vi "Actor Core.vi"(8 "error in":errorcluster, 11 "Network Endpoint":refnum<class "Network Endpoint.lvclass">) -> (0 "error out":errorcluster, 3 "Actor out":refnum<class "Actor.lvclass">)   [LabVIEW 2020, in "Network Endpoint.lvlib" / "Network Endpoint.lvclass"]
doc: "Manages the reader network stream. Waits for a remote writer to connect. Once a connection is established, forwards received messages to its parent node."
uses:
  Network Endpoint.lvclass
  C:/Program Files (x86)/National Instruments/LabVIEW 2020/vi.lib/ActorFramework/Actor/Actor.lvclass
  <vilib>/ActorFramework/Actor/Actor.lvclass
  <vilib>/ActorFramework/Actor/Actor.lvclass/Actor.ctl
  <vilib>/ActorFramework/Message Enqueuer/Message Enqueuer.lvclass/Message Enqueuer.ctl
  Network Endpoint.lvclass/Network Endpoint.ctl
  <vilib>/ActorFramework/Report Error Msg/Report Error Msg.lvclass/Report Error Msg.ctl
  <vilib>/ActorFramework/Message Enqueuer/Init from Existing Queue.vi
  <vilib>/ActorFramework/Report Error Msg/Report Error Msg.lvclass
  C:/Program Files (x86)/National Instruments/LabVIEW 2020/vi.lib/ActorFramework/Message/Message.lvclass
  <vilib>/ActorFramework/Message Priority Queue/Priority Enqueue.vi
  Abstract Classes/Message Stream/Message Stream.lvclass
  <vilib>/ActorFramework/Message Enqueuer/Message Enqueuer.lvclass
  Abstract Classes/Message Flattener/Message Flattener.lvclass
  <resource>/AFDebug/AF Debug.lvlib
  <vilib>/ActorFramework/Message/Message.lvclass
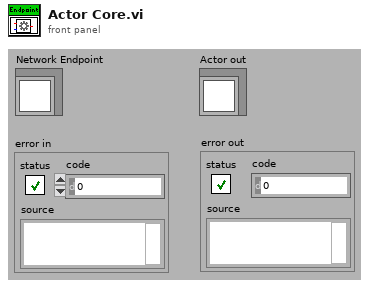
[diagram p1: front panel]
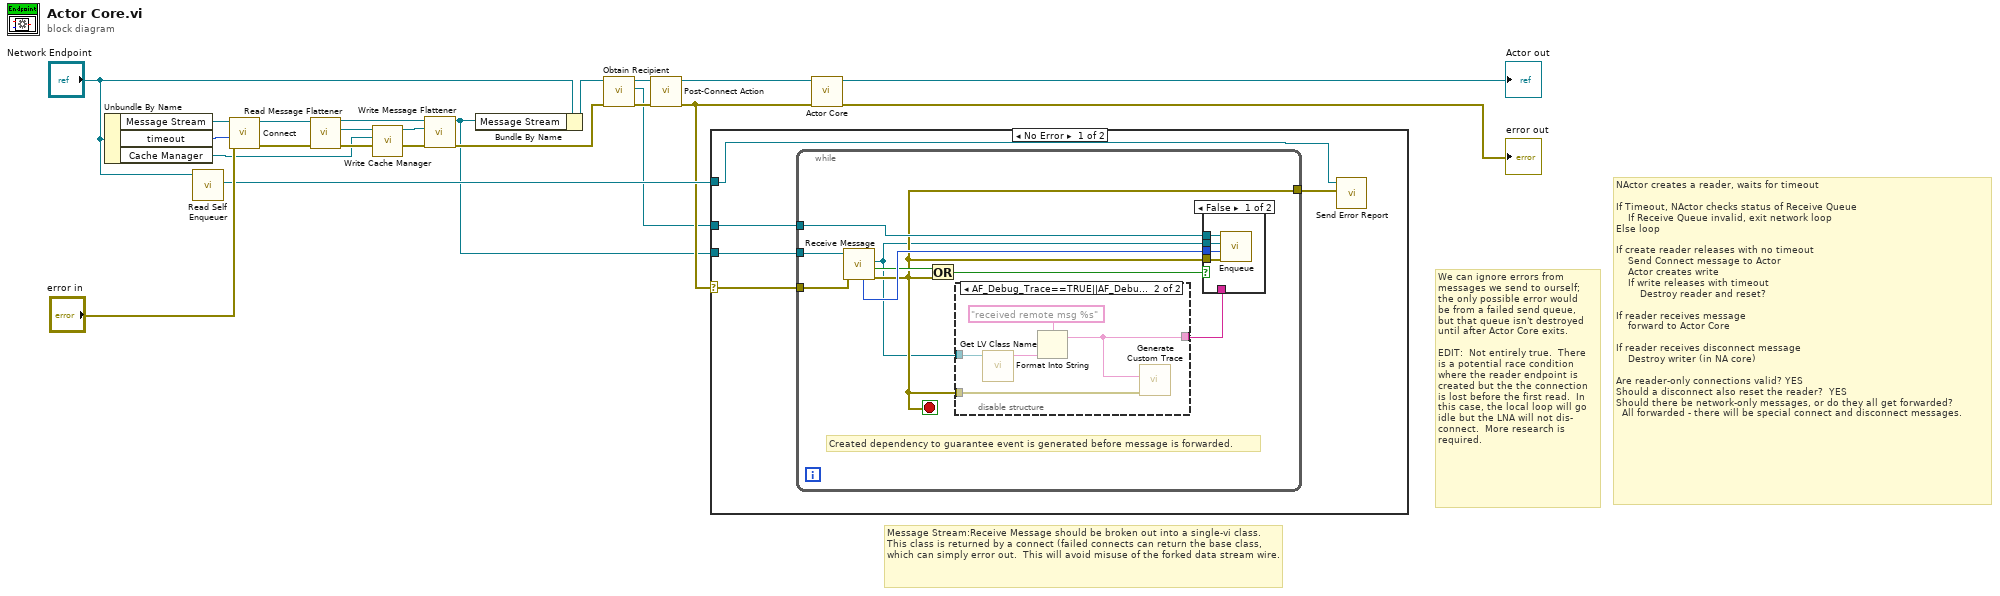
[diagram p0: block diagram]
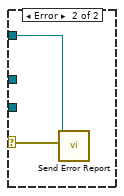
[diagram p4: hidden frame]
diagram:
  # "Message Stream:Receive Message should be broken out into a single-vi class.\nThis class is returned by a connect (failed connects can return the base class, which can simply error out.  This will avoid misuse of the forked data stream wire."
  # "We can ignore errors from\nmessages we send to ourself;\nthe only possible error would\nbe from a failed send queue,\nbut that queue isn't destroyed\nuntil after Actor Core exits.\n\nEDIT:  Not entirely true.  There\nis a potential race condition \nwhere the reader endpoint is\ncreated but the the connection\nis lost before the first read.  In\nthis case, the local loop will go\nidle but the LNA will not dis-\nconnect.  More research is\nrequired."
  # "NActor creates a reader, waits for timeout\n\nIf Timeout, NActor checks status of Receive Queue\n    If Receive Queue invalid, exit network loop\nElse loop\n\nIf create reader releases with no timeout\n    Send Connect message to Actor\n    Actor creates write\n    If write releases with timeout\n        Destroy reader and reset?\n\nIf reader receives message\n    forward to Actor Core\n\nIf reader receives disconnect message\n    Destroy writer (in NA core)\n\nAre reader-only connections valid? YES\nShould a disconnect also reset the reader?  YES\nShould there be network-only messages, or do they all get forwarded?\n  All forwarded - there will be special connect and disconnect messages."
  n1 = Unbundle By Name("Network Endpoint") -> ("Message Stream"=w18:refnum<class "Message Stream.lvclass">, "timeout"=w17:i32, "Cache Manager"=w5:refnum<class "Cache Manager.lvclass">)
  n2 = call <vilib>:"Read Self Enqueuer.vi"("Actor"="Network Endpoint") -> ("Self Enqueuer"=w15:refnum<class "Message Enqueuer.lvclass">)  [unwired: 10 in]
  n3 = call-dynamic "Connect.vi"("error in (no error)"="error in", "timeout"=w17, "Message Stream in"=w18) -> ("error out"=w7:errorcluster, "Message Stream out"=w3:refnum<class "Message Stream.lvclass">)  [unwired: 7 in]
  n4 = call-dynamic "Read Message Flattener.vi"("Message Stream in"=w3) -> ("Message Flattener.lvclass"=w6:refnum<class "Message Flattener.lvclass">, "Message Stream out"=w2:refnum<class "Message Stream.lvclass">)  [unwired: 9 in]
  n5 = call-dynamic "Write Cache Manager.vi"("Cache Manager DVR.lvclass"=w5, "Message Flattener in"=w6) -> ("Message Flattener out"=w4:refnum<class "Message Flattener.lvclass">)  [unwired: 9 in]
  n6 = call-dynamic "Write Message Flattener.vi"("Message Flattener.lvclass"=w4, "Message Stream in"=w2) -> ("Message Stream out"=w1:refnum<class "Message Stream.lvclass">)  [unwired: 9 in]
  n7 = Bundle By Name(cluster="Network Endpoint", "Message Stream"=w1) -> (w10:refnum<class "Network Endpoint.lvclass">)
  n8 = call-dynamic "Obtain Recipient.vi"("error in (no error)"=w7, "Network Endpoint in"=w10) -> ("error out"=w13:errorcluster, "Recipient Enqueuer"=w8:refnum<class "Message Enqueuer.lvclass">, "Network Endpoint out"=w12:refnum<class "Network Endpoint.lvclass">)  [unwired: 7 in]
  n9 = call-dynamic "Post-Connect Action.vi"("error in (no error)"=w13, "Network Endpoint in"=w12) -> ("error out"=w9:errorcluster, "Network Endpoint out"=w11:refnum<class "Network Endpoint.lvclass">)  [unwired: 8 in]
  n10 = case shown="No Error" w9 {
    selector: w9 -> [w25 w45]
    tunnel: w8 -> [w24 _]
    tunnel: w1 -> [w23 _]
    tunnel: w15 -> [w21 w44]
    frame No Error {
      n11 = while {
        tunnel: w25 -> [w33]
        tunnel: w23 -> [w32]
        tunnel: w24 -> [w34]
        tunnel: [w27] -> w22
        stop <- w27 stop-if-true
        # "Created dependency to guarantee event is generated before message is forwarded."
        n12 = call-dynamic "Receive Message.vi"("error in (no error)"=w33, "Message Stream in"=w32) -> ("error out"=w27:errorcluster, "Timed out?"=w30:bool, "Message"=w26:refnum<class "Message.lvclass">, "priority"=w31:i32)  [unwired: 5 in, 1 out]
        n13 = Or(x=w30, y=w27) -> (x .or. y?=w29:bool)
        n14 = disable-structure "Conditional Disable Structure" shown="AF_Debug_Trace==TRUE||AF_Debug_Trace==True" {
          disable-tunnel: w27 -> [_ w43]
          disable-tunnel: w26 -> [_ w40]
          disable-tunnel: [_ w39] -> w28
          frame condition #0 (active) {
          }
          frame condition #1 {
            n15 = call <vilib>:"Get LV Class Name.vi"("object"=w40) -> ("class name"=w41:string)  [unwired: 9 in, 1 out]
            n16 = Format Into String(format string="received remote msg %s", w41) -> (resulting string=w39:string)  [unwired: 2 in, 1 out]
            n17 = call <resource>:"Generate Custom Trace.vi"("error in (no error)"=w43, "Custom Action"=w39) -> ()  [unwired: 10 in]
          }
        }
        n18 = case shown="False" w29 {
          tunnel: w34 -> [w38 _]
          tunnel: w26 -> [w37 _]
          tunnel: w31 -> [w36 _]
          tunnel: w27 -> [w35 _]
          tunnel: w28 -> [_ _]
          frame False {
            n19 = call <vilib>:"Enqueue.vi"("error in (no error)"=w35, "Message Priority (Normal)"=w36, "Message"=w37, "Message Enqueuer in"=w38) -> ()  [unwired: 6 in, 2 out]
          }
          frame True {
          }
        }
      }
      n20 = call <vilib>:"Send Error Report.vi"("Error From Sender"=w22, "Message Enqueuer"=w21) -> ()  [unwired: 9 in, 1 out]
    }
    frame Error {
      n21 = call <vilib>:"Send Error Report.vi"("Error From Sender"=w45, "Message Enqueuer"=w44) -> ()  [unwired: 9 in, 1 out]
    }
  }
  n22 = call-parent "Actor Core.vi"("error in"=w9, "Actor in"=w11) -> ("error out"=→"error out":errorcluster, "Actor out"=→"Actor out":refnum<class "Actor.lvclass">)  [unwired: 8 in]
